vi "config_burst.vi"(0 "VISA resource name":refnum<visa-resource-name>="TRIG", 1 "burst count":i32, 2 "burst period (s)":dbl, 3 "error in (no error)":errorcluster, 4 "molecular delay":dbl) -> (5 "VISA resource name out":refnum<visa-resource-name>, 7 "error out":errorcluster)   [LabVIEW 2012]
doc: "Sets he burst period and the burst count. \n\nSets he burst count. When burst mode is enabled, the DG645 \noutputs burst count delay cycles per trigger.\n\nThe burst period sets the time between delay cycles during a burst. \nThe burst period may range from 100 ns to 2000 – 10 ns in 10 ns steps."
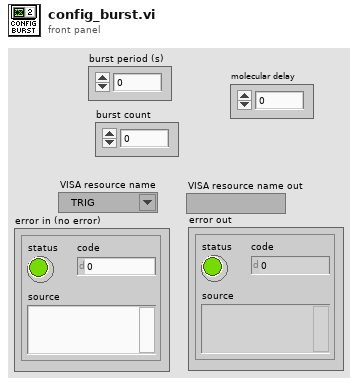
[diagram p1: front panel]
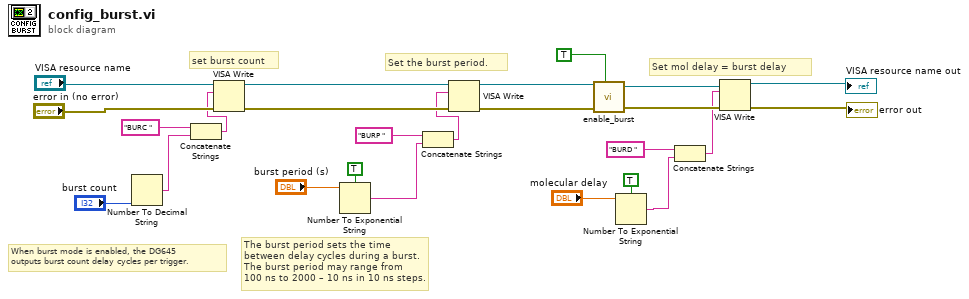
[diagram p0: block diagram]
diagram:
  # "Set mol delay = burst delay"
  # "Set the burst period."
  # "When burst mode is enabled, the DG645 \noutputs burst count delay cycles per trigger."
  # "The burst period sets the time \nbetween delay cycles during a burst. \nThe burst period may range from \n100 ns to 2000 – 10 ns in 10 ns steps."
  # "set burst count"
  n1 = Number To Decimal String(number="burst count") -> (decimal integer string=w17:string)  [unwired: 1 in]
  n2 = Concatenate Strings("BURC " ("Query 2"), w17) -> (w21:string)
  n3 = VISA Write(VISA resource name="VISA resource name", write buffer=w21, error in (no error)="error in (no error)") -> (VISA resource name out=w19:refnum<visa-resource-name>, error out=w22:errorcluster)  [unwired: 1 out]
  n4 = Number To Exponential String(number="burst period (s)", 1:TRUE ("use system decimal point (T)")) -> (E-format string=w15:string)  [unwired: 2 in]
  n5 = Concatenate Strings("BURP " ("Query 2"), w15) -> (w18:string)
  n6 = VISA Write(VISA resource name=w19, write buffer=w18, error in (no error)=w22) -> (VISA resource name out=w11:refnum<visa-resource-name>, error out=w12:errorcluster)  [unwired: 1 out]
  n7 = call "enable_burst.vi"("VISA resource name"=w11, "error in (no error)"=w12, "Burst enable?"=TRUE) -> ("VISA resource name out"=w8:refnum<visa-resource-name>, "error out"=w10:errorcluster)  [unwired: 3 in]
  n8 = Number To Exponential String(number="molecular delay", 1:TRUE ("use system decimal point (T)")) -> (E-format string=w3:string)  [unwired: 2 in]
  n9 = Concatenate Strings("BURD " ("Query 2"), w3) -> (w2:string)
  n10 = VISA Write(VISA resource name=w8, write buffer=w2, error in (no error)=w10) -> (VISA resource name out=→"VISA resource name out":refnum<visa-resource-name>, error out=→"error out":errorcluster)  [unwired: 1 out]
